vi "Initialize Embedded Data Logger Custom Device.vi"(8 "error in":errorcluster, 11 "embedded data logger in":T1 format="%.0x") -> (0 "error out":errorcluster, 3 "embedded data logger out":T1 format="%.0x")   [LabVIEW 2027, in "Embedded Data Logger Scripting.lvlib"]
uses:
  Embedded Data Logger Scripting.lvlib
  <vilib>/NI VeriStand/Custom Device API/Custom Device Item Ref.ctl
  <vilib>/NI VeriStand/Custom Device API/Custom Device Channel Type.ctl
  <vilib>/NI VeriStand/Custom Device API/Custom Device Channel.ctl
  <vilib>/NI VeriStand/Custom Device API/Custom Device API.lvlib
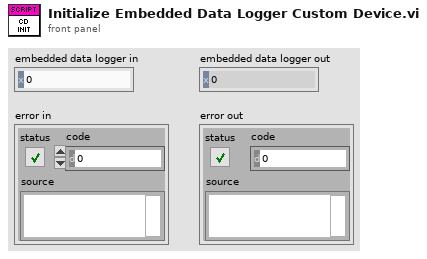
[diagram p1: front panel]
types:
  T1 = typedef "Custom Device API.lvlib/Custom Device Item Ref.ctl" = u64
  T2 = typedef "Custom Device API.lvlib/Custom Device Channel Type.ctl" = enum16{"Input", "Output"}
  T3 = typedef "Custom Device API.lvlib/Custom Device Channel.ctl" = cluster{"Type":T2, "Units":string, "Default Value":dbl, "Faultable":bool, "Scalable":bool}
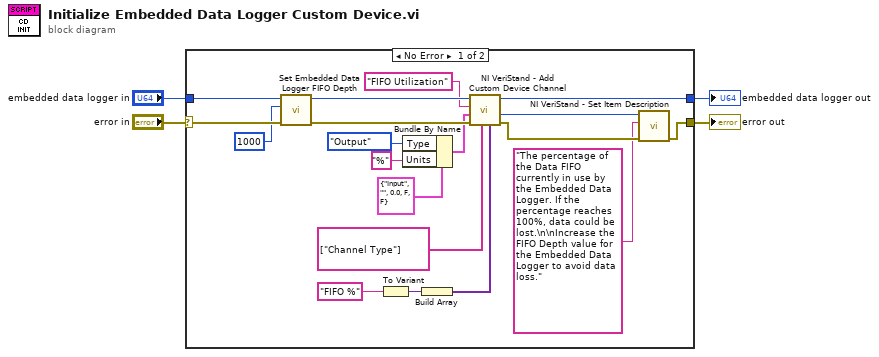
[diagram p0: block diagram]
diagram:
  n1 = case shown="No Error" "error in" {
    selector: "error in" -> [w22 w25]
    tunnel: [w5 w25] -> w1
    tunnel: [w18 w24] -> w3
    tunnel: "embedded data logger in" -> [w23 w24]
    frame No Error {
      n2 = call "Set Embedded Data Logger FIFO Depth.vi"("error in"=w22, "fifo depth"=1000 ("Value"), "embedded data logger in"=w23) -> ("error out"=w19:errorcluster, "embedded data logger out"=w20:T1)  [unwired: 7 in]
      n3 = To Variant(anything="FIFO %" ("String")) -> (Variant=w10:variant)
      n4 = Bundle By Name(cluster=T3 {"Type"=enum."Input", "Units"="", "Default Value"=0.0, "Faultable"=FALSE, "Scalable"=FALSE} ("Channel"), "Type"=Custom_Device_Channel_Type."Output", "Units"="%") -> (w15:T3)
      n5 = Build Array(w10) -> (w9:variant[])
      n6 = call <vilib>:"NI VeriStand - Add Custom Device Channel.vi"("Property Values"=w9, "Property names"=string[] ["Channel Type"], "error in (no error)"=w19, "Channel"=w15, "Channel Name"="FIFO Utilization", "Parent Ref in"=w20) -> ("error out"=w7:errorcluster, "Channel Ref"=w8:T1, "Parent Ref out"=w18:T1)  [unwired: 2 in, 1 out]
      n7 = call <vilib>:"NI VeriStand - Set Item Description.vi"("error in (no error)"=w7, "Description"="The percentage of the Data FIFO currently in use by the Embedded Data Logger. If the percentage reaches 100%, data could be lost.\n\nIncrease the FIFO Depth value for the Embedded Data Logger to avoid data loss.", "Item Ref in"=w8) -> ("error out"=w5:errorcluster)  [unwired: 6 in, 2 out]
    }
    frame Error {
    }
  }
  "embedded data logger out" <- w3
  "error out" <- w1
